vi "analyze_test_data.vi"() -> ()   [LabVIEW 2021]
uses:
  <vilib>/Waveform/WDTFileIO.llb/Read Waveform from File.vi
panel:
  out "Waveform Graph":waveform(dbl)(graph)
  out "normalized waveform":waveform(dbl)
  out "Waveform":waveform(dbl)
  out "filtered waveform":waveform(dbl)(graph)
  out "data points in waveform":i32
  out "first waveform in array (raw)":waveform(dbl)(graph)
  out "amount of waveforms in file":i32
  out "element":waveform(dbl)
  out "all waveforms in record":waveform(dbl)[](array[waveform])
  out "error out":errorcluster
  in  "file path (use dialog)":path
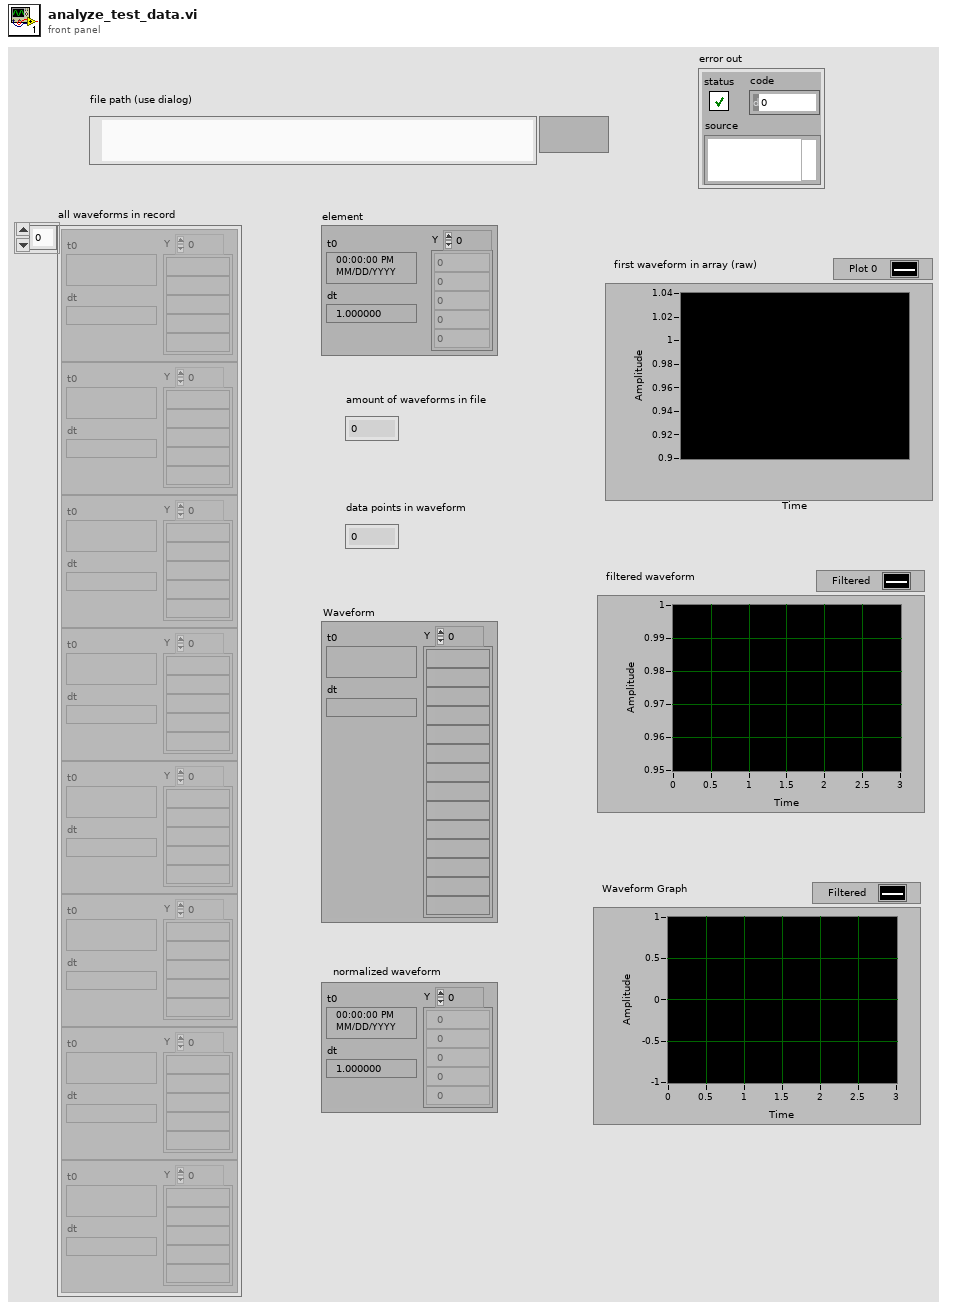
[diagram p1: front panel]
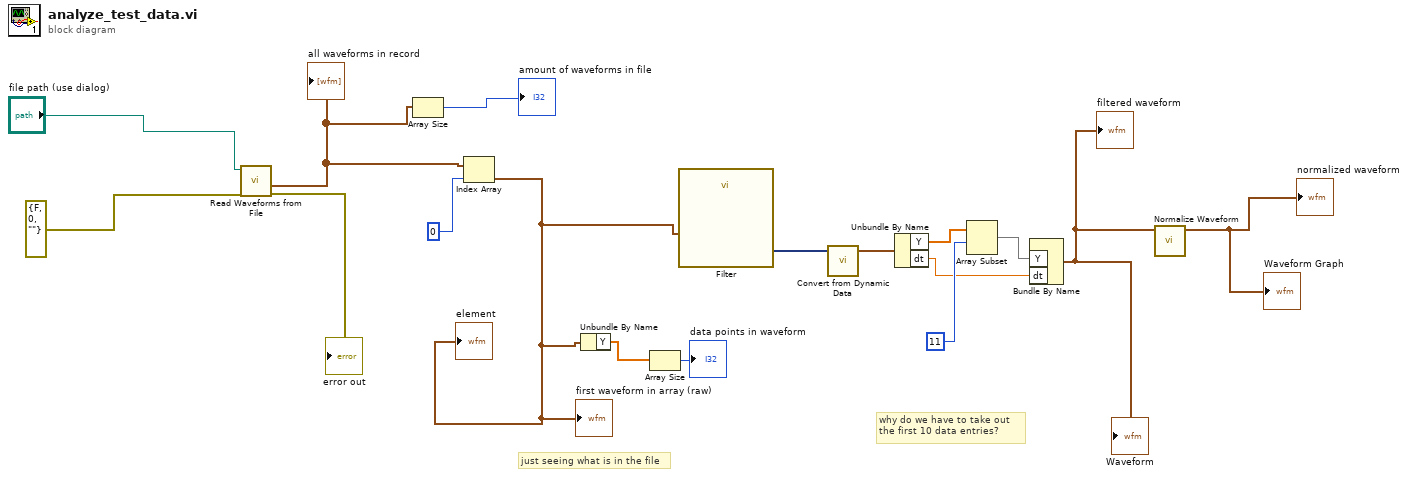
[diagram p0: block diagram]
diagram:
  # "why do we have to take out\nthe first 10 data entries?"
  # "just seeing what is in the file"
  n1 = call-poly <vilib>:"Read Waveforms from File.vi"("error in (no error)"=errorcluster {"status"=FALSE, "code"=0, "source"=""} ("error in"), "file path (dialog if empty)"="file path (use dialog)") -> ("error out"=→"error out":errorcluster, "all waveforms in record"=w13:waveform(dbl)[])  [unwired: 4 in, 2 out]
  "all waveforms in record" <- w13
  n2 = Array Size(array=w13) -> (size(s)=→"amount of waveforms in file":i32)
  n3 = Index Array(array=w13, index=0) -> (element=w9:waveform(dbl))
  "element" <- w9
  "first waveform in array (raw)" <- w9
  n4 = Unbundle By Name(w9) -> ("Y"=w11:dbl[])
  n5 = Array Size(array=w11) -> (size(s)=→"data points in waveform":i32)
  n6 = call "Filter"("Signal"=w9) -> ("Filtered Signal"=w8:dynamicdata)  [unwired: 9 in, 1 out]
  n7 = call "Convert from Dynamic Data"("Dynamic Data Type"=w8) -> ("Waveform"=w6:waveform(dbl))  [unwired: 3 in]
  n8 = Unbundle By Name(w6) -> ("Y"=w5:dbl[], "dt"=w2:dbl)
  n9 = Array Subset(array=w5, index=11) -> (w3:dbl[])  [unwired: 1 in]
  n10 = Bundle By Name("Y"=w3, "dt"=w2) -> (w1:waveform(dbl))  [unwired: 1 in]
  "filtered waveform" <- w1
  "Waveform" <- w1
  n11 = call <vilib>:"Normalize Waveform.vi"("waveform in"=w1) -> ("normalized waveform"=→"normalized waveform" →"Waveform Graph":waveform(dbl))  [unwired: 7 in, 3 out]
